vi "Example-date-time-fomat.vi"() -> ()   [LabVIEW 2012]
panel:
  out "date/time-string":string
  in  "Instrument Name":string="Instrument-name-"
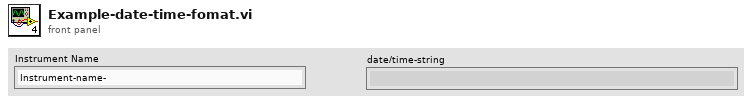
[diagram p1: front panel]
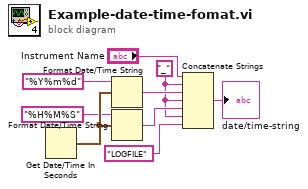
[diagram p0: block diagram]
diagram:
  w3 = "_" ("string")
  n1 = Get Date/Time In Seconds() -> (seconds since 1Jan1904=w8:timestamp)
  n2 = Format Date/Time String(time format string (%c)="%Y%m%d", seconds (now)=w8) -> (date/time string=w6:string)  [unwired: 1 in]
  n3 = Format Date/Time String(time format string (%c)="%H%M%S", seconds (now)=w8) -> (date/time string=w7:string)  [unwired: 1 in]
  n4 = Concatenate Strings("Instrument Name", w3, w6, w3, w7, w3, "LOGFILE" ("pattern")) -> (→"date/time-string":string)
